vi "Log Error.vi"(7 "Level":T1, 8 "error in (no error)":errorcluster) -> (0 "error out":errorcluster)   [LabVIEW 2016, in "Stream Log.lvlib" / "Global Application Log.lvclass"]
doc: "--\nCopyright © 2017 Composed SystemsI All rights reserved.\n\nAuthor: Jon McBee <jon.mcbee@composed.io>\n\nThis library is provided \"AS IS\" ,WITHOUT WARRANTIES OR\nCONDITIONS OF ANY KIND, either express or implied.\n\nComposed Systems -- composed.io\n\nStream 0.0.1.1\nJon McBee - Composed Systems\nCopyright (c) 2017, Composed Systems"
uses:
  <userlib>/Composed Systems/Stream/Log/Global Application Log/Global Application Log.lvclass
  <userlib>/Composed Systems/Stream/Log/Application Log/Log Level.ctl
  <userlib>/Composed Systems/Stream/Log/Global Application Log/Global Application Log.lvclass/Global Application Log.ctl
  <userlib>/Composed Systems/Stream/Log/Application Log/Application Log.lvclass
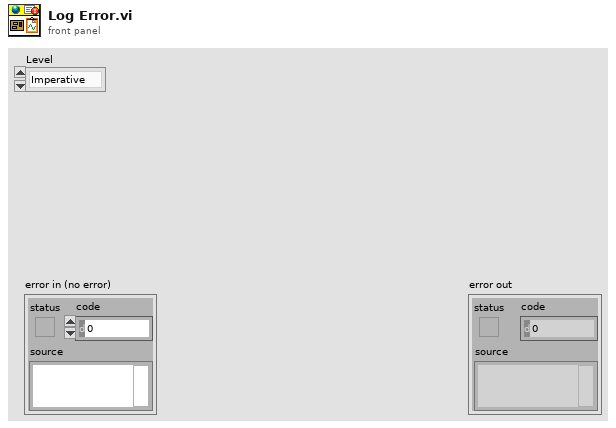
[diagram p1: front panel]
types:
  T1 = typedef "Stream Log.lvlib/Application Log.lvclass/Log Level.ctl" = enum16{"Imperative", "Major", "Minor", "Debug", "Off"}
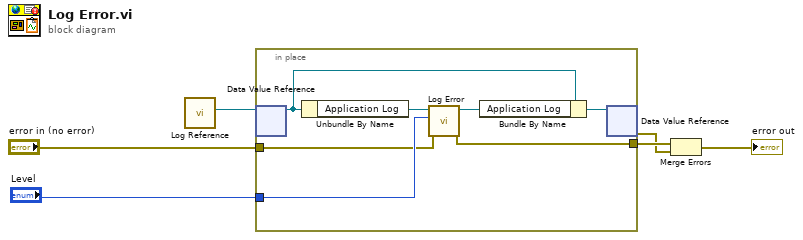
[diagram p0: block diagram]
diagram:
  n1 = call <userlib>:"Log Reference.vi"() -> ("Global Log Reference out"=w4:refnum<data-value>)  [unwired: 11 in]
  n2 = in-place {
    in-place-border: "Level" -> [w8]
    in-place-border: [w9] -> w3
    in-place-border: "error in (no error)" -> [w7]
    n3 = in-place-dvr #1(w4) -> (w13:refnum<class "Global Application Log.lvclass">)  [unwired: 1 out]
    n4 = Unbundle By Name(w13) -> ("Application Log"=w11:refnum<class "Application Log.lvclass">)
    n5 = call <userlib>:"Log Error.vi"("error in (no error)"=w7, "Level"=w8, "Application Log in"=w11) -> ("error out"=w9:errorcluster, "Application Log out"=w10:refnum<class "Application Log.lvclass">)  [unwired: 6 in, 1 out]
    n6 = Bundle By Name(cluster=w13, "Application Log"=w10) -> (w12:refnum<class "Global Application Log.lvclass">)
    n7 = in-place-dvr #1(w12) -> (w2:errorcluster)  [unwired: 1 out]
  }
  n8 = Merge Errors(w3, w2) -> (→"error out":errorcluster)
